vi "RS232.vi"(8 "error in":errorcluster, 10 "command":string, 11 "RS232_Input":refnum<visa-resource-name>) -> (0 "error out":errorcluster, 2 "response":string, 3 "RS232_Output":refnum<visa-resource-name>)   [LabVIEW 2017]
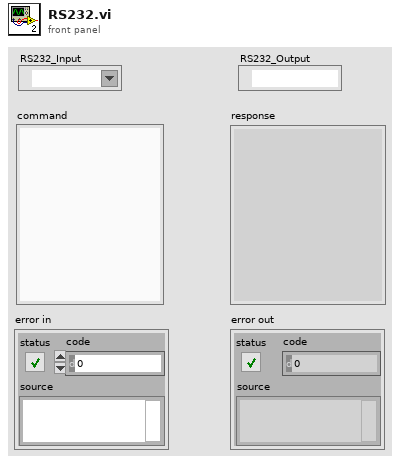
[diagram p1: front panel]
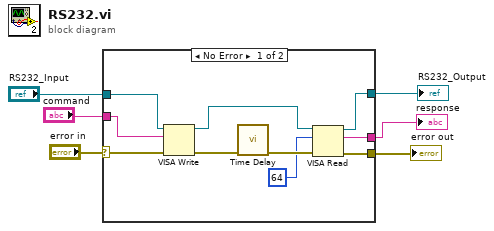
[diagram p0: block diagram]
diagram:
  n1 = case shown="No Error" "error in" {
    selector: "error in" -> [w16 w18]
    tunnel: "RS232_Input" -> [w15 w19]
    tunnel: "command" -> [w14 w17]
    tunnel: [w9 w18] -> w3
    tunnel: [w8 w19] -> w2
    tunnel: [w7 w17] -> w1
    frame No Error {
      n2 = VISA Write(VISA resource name=w15, write buffer=w14, error in (no error)=w16) -> (VISA resource name out=w11:refnum<visa-resource-name>, error out=w13:errorcluster)  [unwired: 1 out]
      n3 = call "Time Delay"("error in (no error)"=w13) -> ("error out"=w12:errorcluster)  [unwired: 10 in]
      n4 = VISA Read(VISA resource name=w11, byte count=u32 64, error in (no error)=w12) -> (VISA resource name out=w8:refnum<visa-resource-name>, read buffer=w7:string, error out=w9:errorcluster)  [unwired: 1 out]
    }
    frame Error {
    }
  }
  "error out" <- w3
  "RS232_Output" <- w2
  "response" <- w1
